vi "GVSResize Panel Child For Load.vi"(8 "spliter array":refnum<vi>[](array[refnum]), 9 "SubPanel array":refnum<vi>[](array[refnum]), 10 "DataView Array Idx":i32) -> ()   [LabVIEW 2013]
uses:
  GVSNew View Global.vi
panel:
  in  "cur_sp_hei":i32
  in  "cur_sp_wid":i32
  in  "cur_sp_ypos":i32
  in  "cur_sp_xpos":i32
  in  "sp_mUp_hei":i32
  in  "sp_mUp_wid":i32
  in  "sp_mUp_ypos":i32
  in  "sp_mUp_xpos":i32
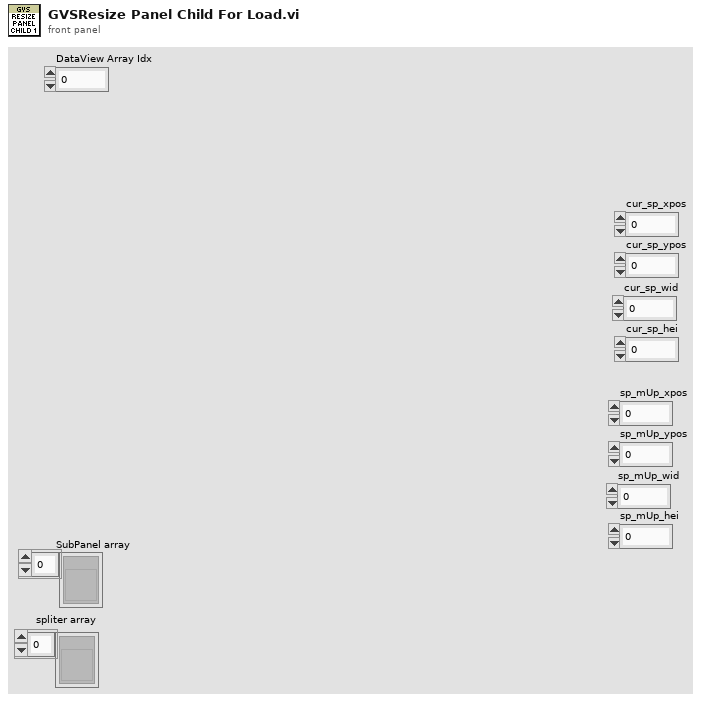
[diagram p1: front panel]
types:
  T1 = typedef "Graph Main Info Cluster.ctl" = cluster{"Selected_BarIdx":i32, "Selected_PanelIdx":i32, "Graph Main VIRef":refnum<vi>, "ToolBarClick":bool, "Spliter Ref Array":refnum<vi>[], "Panel Ref Array":refnum<vi>[], "Spliter_matrix":i32[][], "Panel_matrix":i32[][], "child_spliterIdx_matrix":i32[][], "split_pos_matrix":i32[][], "Title State":bool, "sQueueName":string, "Frame nID":i32, "Graph VIRef Array":cluster{"Graph VIRef":refnum<vi>, "Panel Idx":i32, "Frame VIRef":refnum<vi>, "Icon Ring":i32, "Graph Type":string}[], "View Type":string}
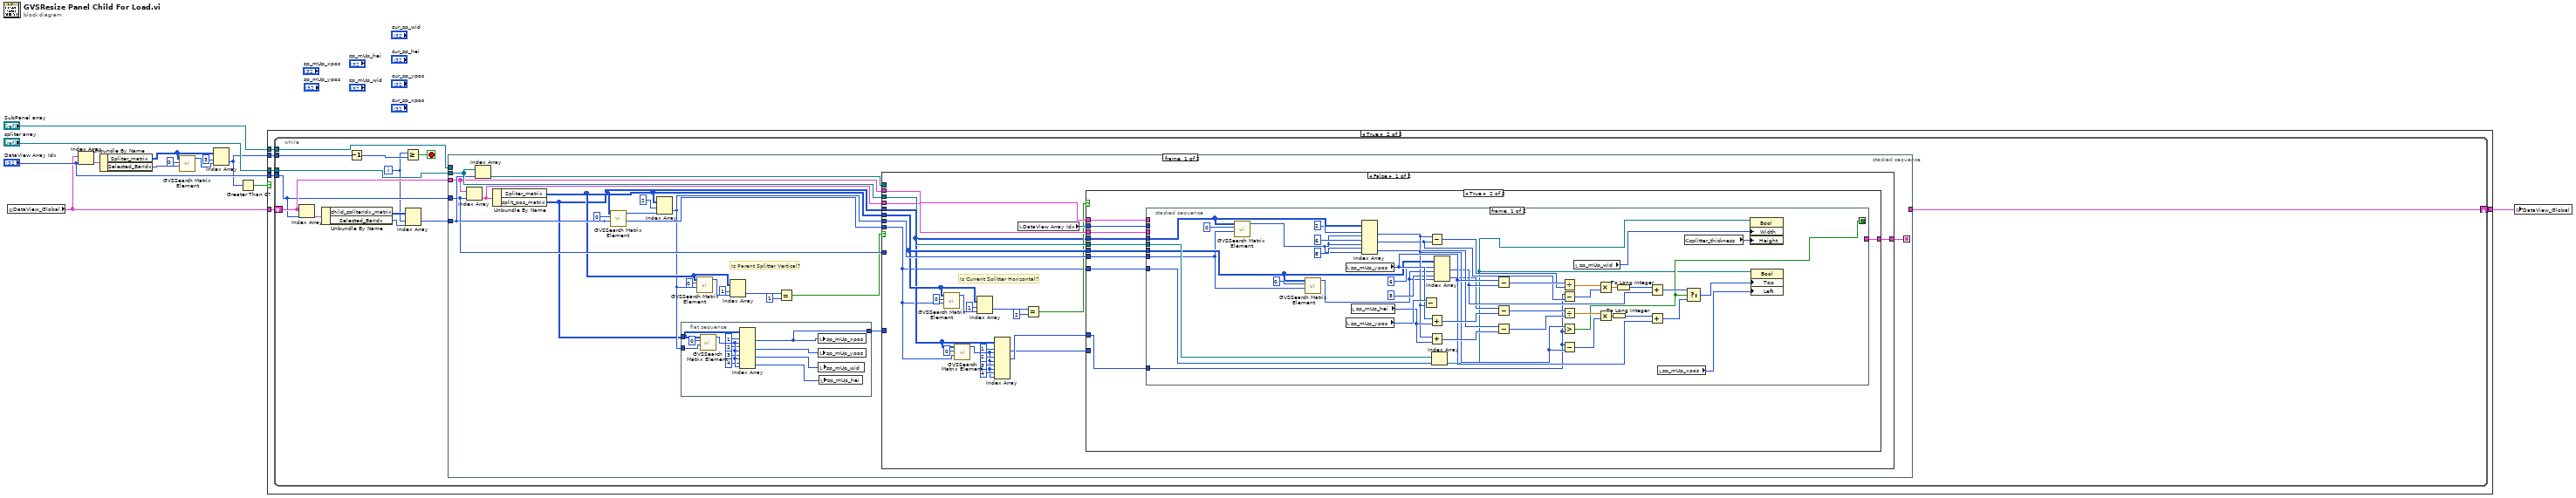
[diagram p0: block diagram]
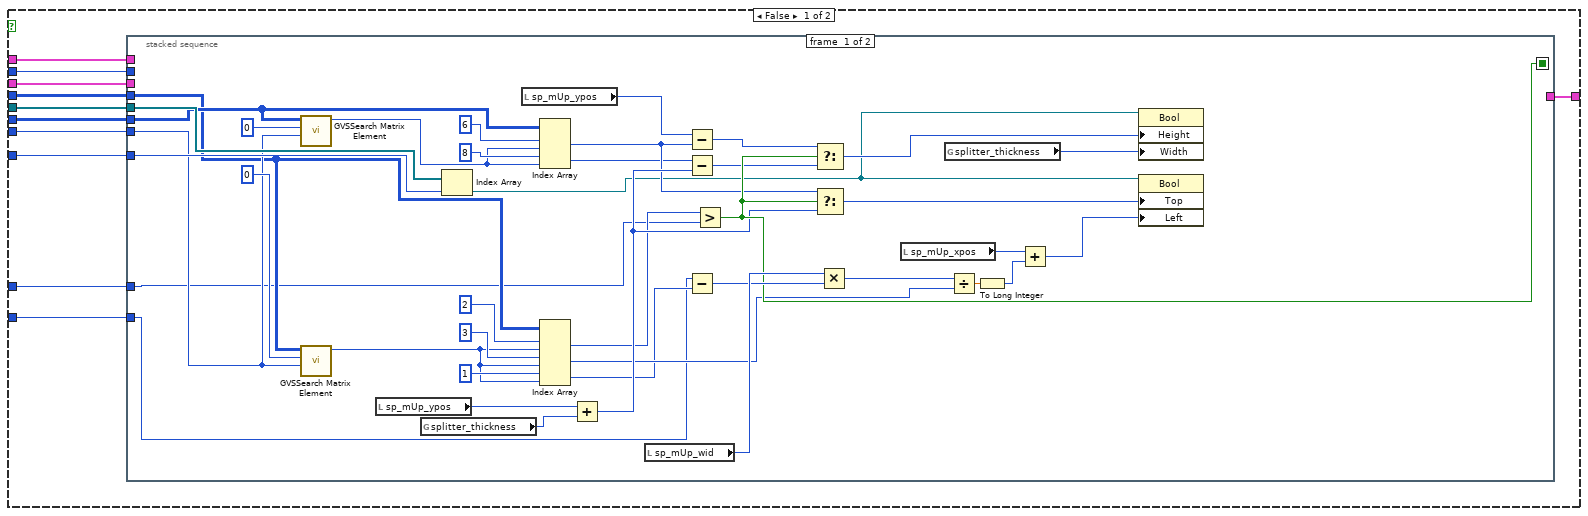
[diagram p3: hidden frame]
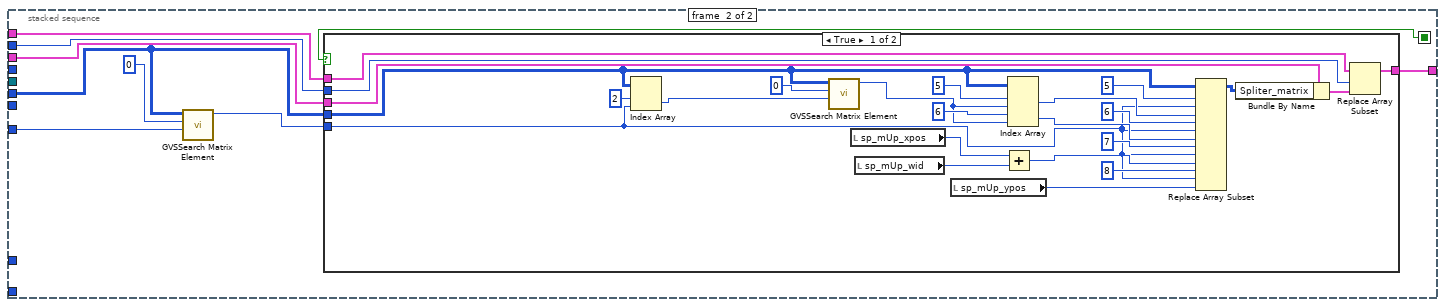
[diagram p4: hidden frame]
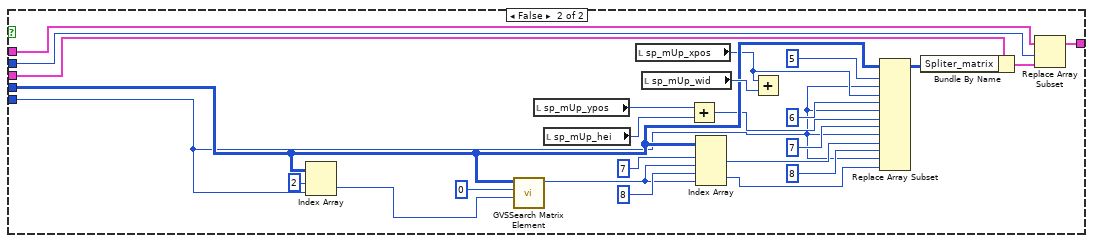
[diagram p5: hidden frame]
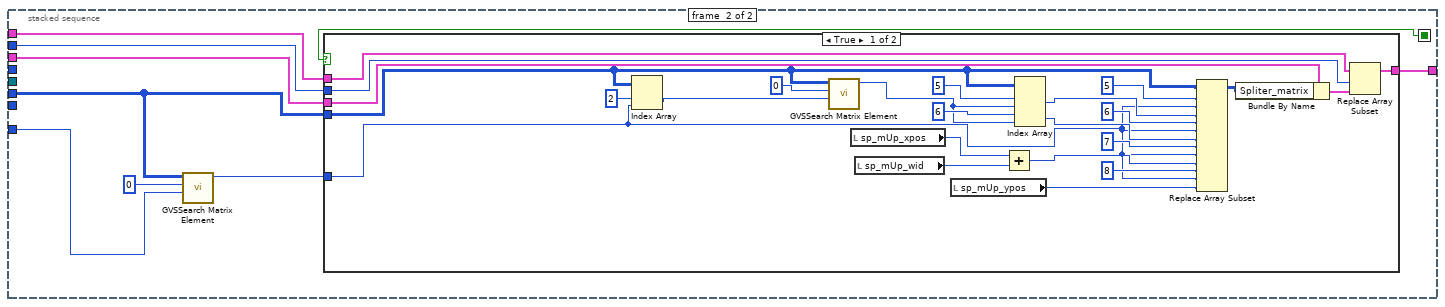
[diagram p6: hidden frame]
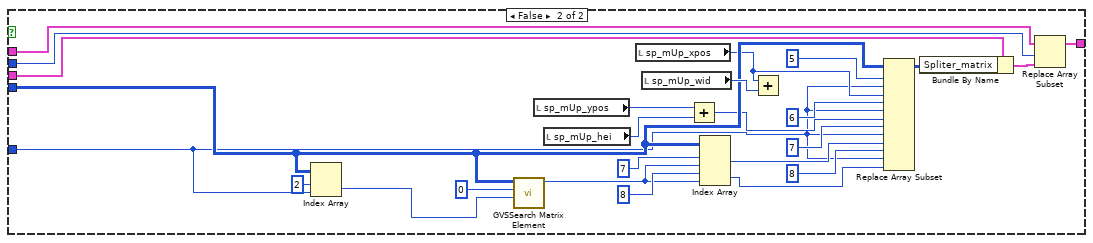
[diagram p7: hidden frame]
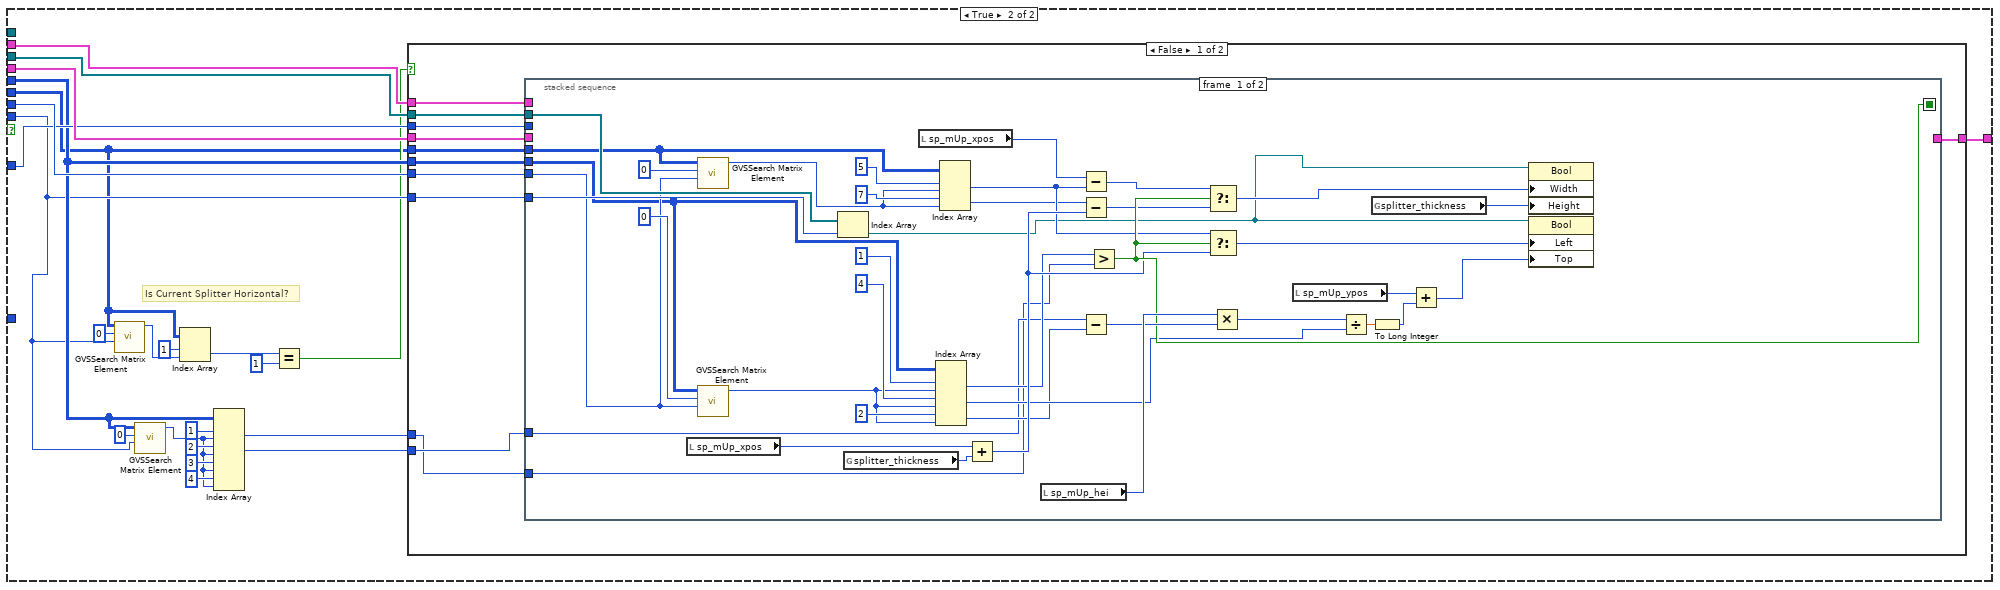
[diagram p8: hidden frame]
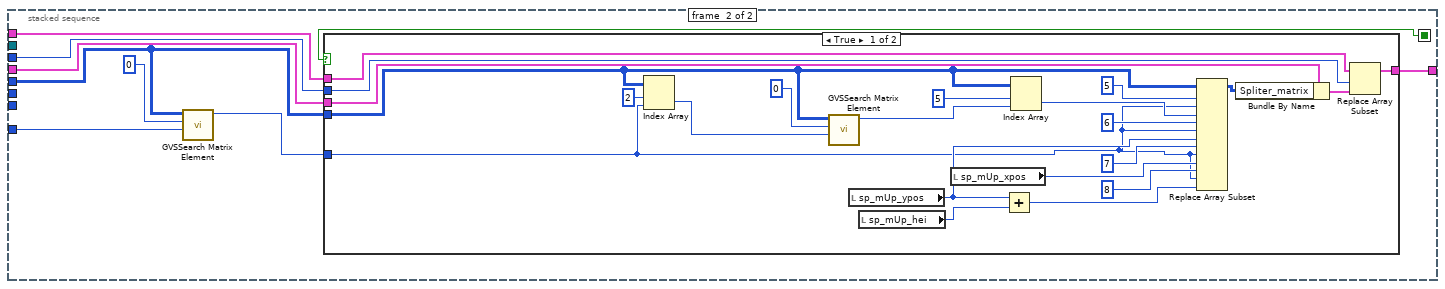
[diagram p9: hidden frame]
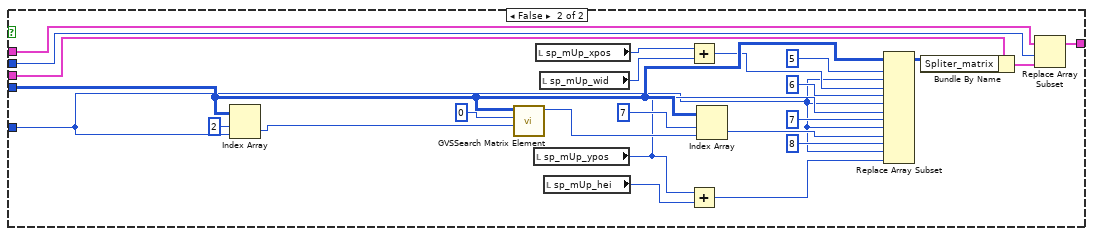
[diagram p10: hidden frame]
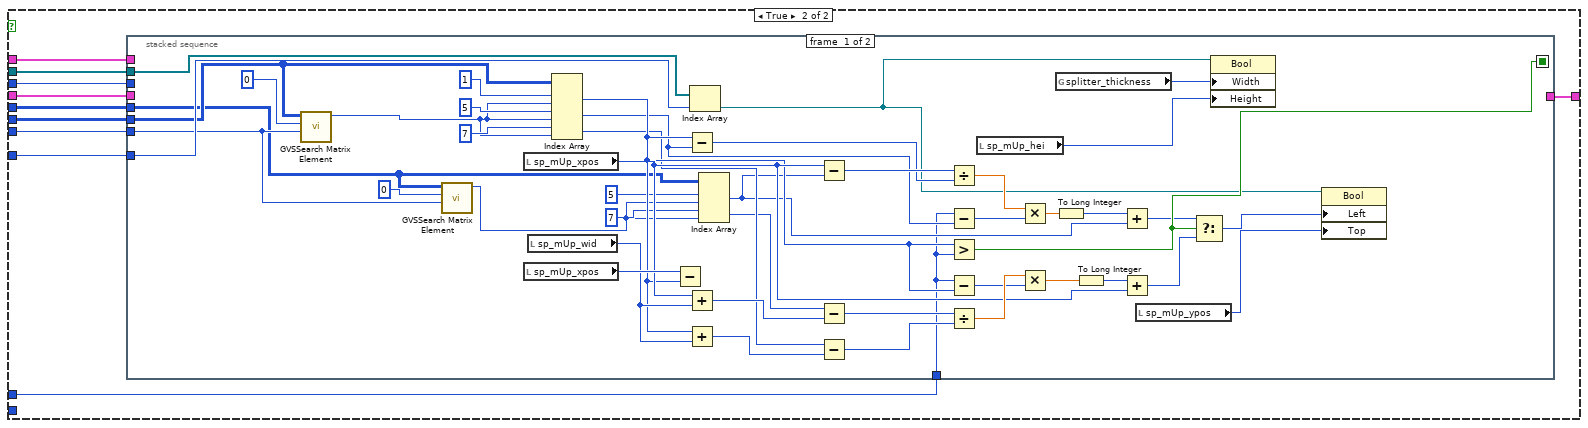
[diagram p11: hidden frame]
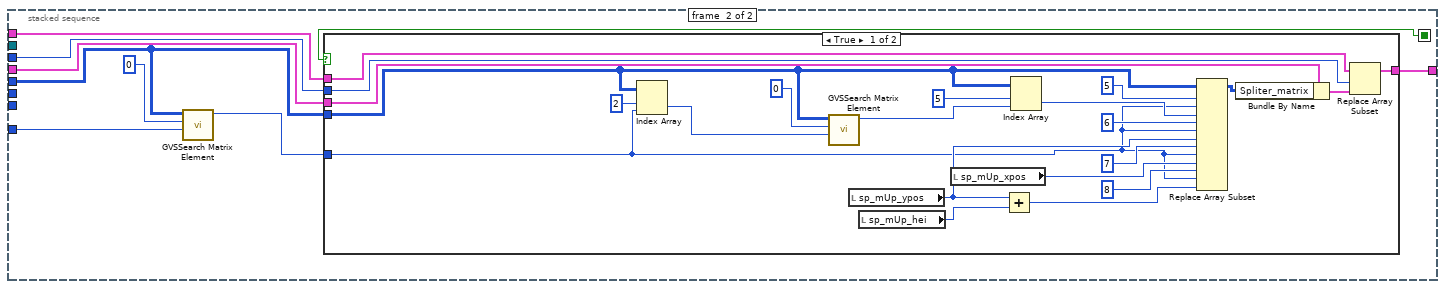
[diagram p12: hidden frame]
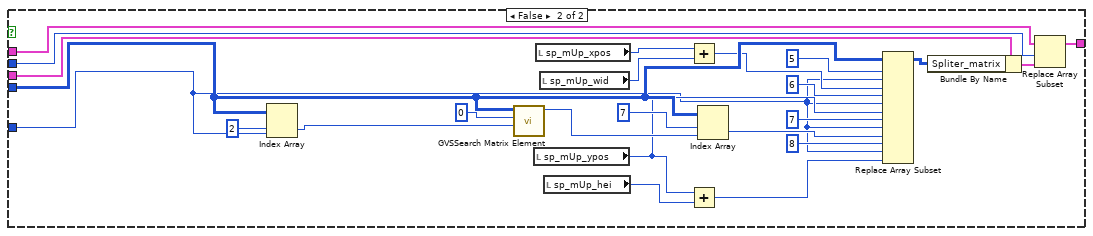
[diagram p13: hidden frame]
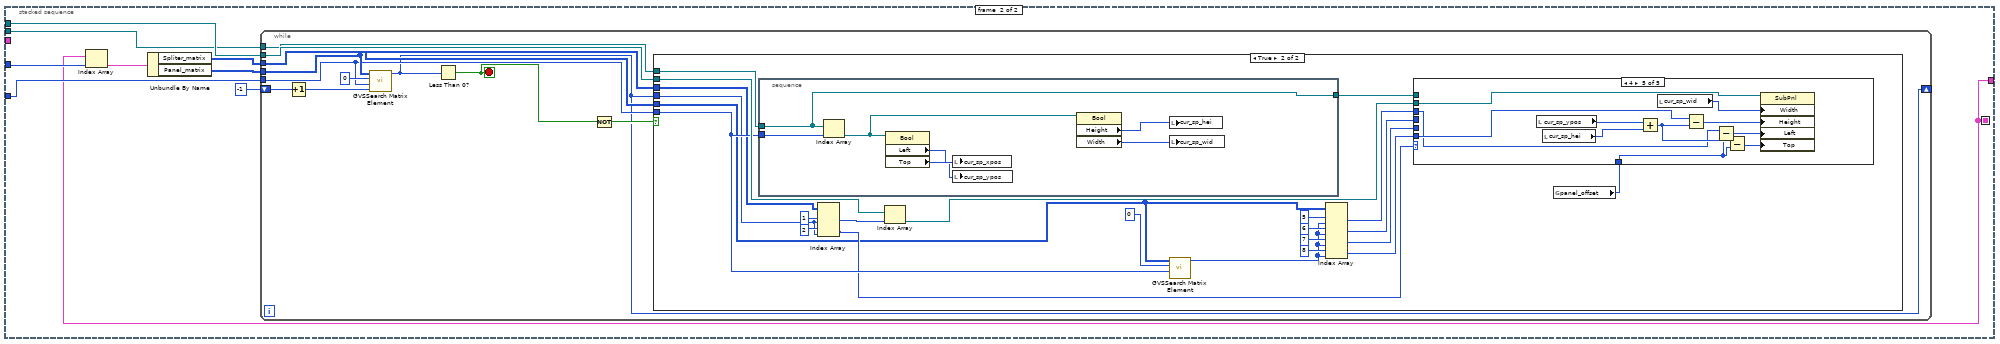
[diagram p14: hidden frame]
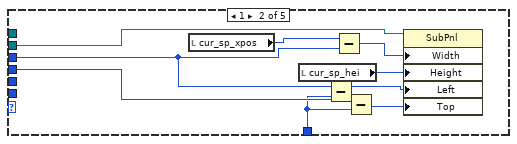
[diagram p17: hidden frame]
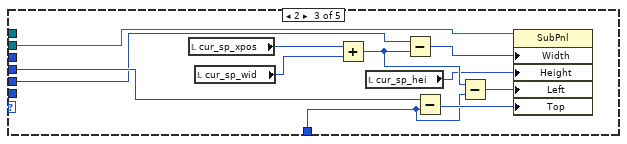
[diagram p18: hidden frame]
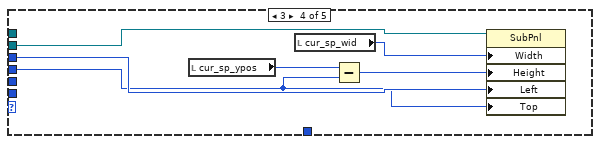
[diagram p19: hidden frame]
diagram:
  n1 = global read "GVSNew View Global.vi" "DataView_Global"() -> (w7:T1[])
  n2 = Index Array(array=w7, index="DataView Array Idx") -> (element=w10:T1)
  n3 = Unbundle By Name(w10) -> ("Spliter_matrix"=w4:i32[][], "Selected_BarIdx"=w9:i32)
  n4 = call "GVSSearch Matrix Element.vi"("element"=w9, "index (row)"=0, "matrix in"=w4) -> ("index of element"=w2:i32)  [unwired: 8 in]
  n5 = Index Array(array=w4, index (row)=3, index (col)=w2) -> (element=w1:i32)
  n6 = Greater Than 0?(x=w1) -> (x > 0?=w5:bool)
  n7 = case shown="True" w5 {
    tunnel: "spliter array" -> [_ w20]
    tunnel: "SubPanel array" -> [_ w19]
    tunnel: "DataView Array Idx" -> [_ w18]
    tunnel: w1 -> [_ w17]
    tunnel: w7 -> [w14 w16]
    tunnel: [w14 w15] -> w6
    frame False {
    }
    frame True {
      n8 = while {
        tunnel: w20 -> [w31]
        tunnel: w17 -> [w25]
        tunnel: w19 -> [w30]
        tunnel: w18 -> [w26]
        shift-right: [w27] -> w15
        shift-left: w16 -> [w28]
        i -> [w23]
        stop <- w32 stop-if-true
        n9 = Index Array(array=w28, index=w26) -> (element=w29:T1)
        n10 = Unbundle By Name(w29) -> ("child_spliterIdx_matrix"=w24:i32[][], "Selected_BarIdx"=w22:i32)
        n11 = Decrement(x=w25) -> (x-1=w33:i32)
        n12 = Greater Or Equal?(x=w23, y=w33) -> (x >= y?=w32:bool)
        n13 = Index Array(array=w24, index (row)=w23, index (col)=w22) -> (element=w21:i32)
        n14 = stacked-sequence {
          seq-local: [w47 _] -> [_ w548]
          tunnel: w31 -> [w52 w554]
          tunnel: w21 -> [w49 w556]
          tunnel: w30 -> [_ w555]
          tunnel: w26 -> [w46 w551]
          tunnel: w28 -> [w48 _]
          tunnel: [_ w548] -> w27
          frame #0 {
            # "Is Parent Splitter Vertical?"
            n15 = Index Array(array=w48, index=w46) -> (element=w51:T1)
            n16 = Index Array(array=w52, index=w49) -> (element=w53:refnum<vi>)
            n17 = Unbundle By Name(w51) -> ("Spliter_matrix"=w42:i32[][], "split_pos_matrix"=w35:i32[][])
            n18 = call "GVSSearch Matrix Element.vi"("element"=w49, "index (row)"=0, "matrix in"=w42) -> ("index of element"=w44:i32)  [unwired: 8 in]
            n19 = Index Array(array=w42, index (row)=2, index (col)=w44) -> (element=w36:i32)
            n20 = flat-sequence {
              tunnel: w36 -> [w64]
              tunnel: w35 -> [w55]
              tunnel: [w54] -> w34
              frame #0 {
                n21 = call "GVSSearch Matrix Element.vi"("element"=w64, "index (row)"=0, "matrix in"=w55) -> ("index of element"=w63:i32)  [unwired: 8 in]
                n22 = Index Array(array=w55, index (row) #1=1 ("disabled index (row)"), index (col) #1=w63, index (row) #2=2 ("disabled index (row)"), index (col) #2=w63, index (row) #3=3 ("disabled index (row)"), index (col) #3=w63, index (row) #4=4 ("disabled index (row)"), index (col) #4=w63) -> (element #1=w54:i32, element #2=w58:i32, element #3=w57:i32, element #4=w56:i32)
                n23 = local write "sp_mUp_xpos"(w54) -> ()
                n24 = local write "sp_mUp_ypos"(w58) -> ()
                n25 = local write "sp_mUp_wid"(w57) -> ()
                n26 = local write "sp_mUp_hei"(w56) -> ()
              }
            }
            n27 = call "GVSSearch Matrix Element.vi"("element"=w36, "index (row)"=0, "matrix in"=w42) -> ("index of element"=w37:i32)  [unwired: 8 in]
            n28 = Index Array(array=w42, index (row)=1 ("disabled index (row)"), index (col)=w37) -> (element=w40:i32)
            n29 = Equal?(x=w40, y=1) -> (x = y?=w38:bool)
            n30 = case shown="False" w38 {
              tunnel: w53 -> [_ _]
              tunnel: w36 -> [w88 w332]
              tunnel: w52 -> [w87 w331]
              tunnel: w49 -> [w66 w314]
              tunnel: w35 -> [w69 w315]
              tunnel: w42 -> [w77 w310]
              tunnel: w51 -> [w86 w330]
              tunnel: w48 -> [w84 w329]
              tunnel: [w83 w328] -> w47
              tunnel: w46 -> [_ w327]
              tunnel: w34 -> [_ _]
              frame False {
                # "Is Current Splitter Horizontal?"
                n31 = call "GVSSearch Matrix Element.vi"("element"=w66, "index (row)"=0, "matrix in"=w77) -> ("index of element"=w82:i32)  [unwired: 8 in]
                n32 = call "GVSSearch Matrix Element.vi"("element"=w66, "index (row)"=0, "matrix in"=w69) -> ("index of element"=w71:i32)  [unwired: 8 in]
                n33 = Index Array(array=w77, index (row)=1 ("disabled index (row)"), index (col)=w82) -> (element=w80:i32)
                n34 = Index Array(array=w69, index (row) #1=1 ("disabled index (row)"), index (col) #1=w71, index (row) #2=2 ("disabled index (row)"), index (col) #2=w71, index (row) #3=3 ("disabled index (row)"), index (col) #3=w71, index (row) #4=4 ("disabled index (row)"), index (col) #4=w71) -> (element #1=w67:i32, element #2=w68:i32)  [unwired: 2 out]
                n35 = local read "DataView Array Idx"() -> (w85:i32)
                n36 = Equal?(x=w80, y=2) -> (x = y?=w76:bool)
                n37 = case shown="True" w76 {
                  tunnel: w88 -> [w97 w204]
                  tunnel: w87 -> [w99 w205]
                  tunnel: w66 -> [w98 w206]
                  tunnel: w69 -> [w96 w203]
                  tunnel: w77 -> [w95 w202]
                  tunnel: w86 -> [w94 w201]
                  tunnel: w85 -> [w93 w200]
                  tunnel: w84 -> [w92 w199]
                  tunnel: [w91 w198] -> w83
                  tunnel: w68 -> [w90 w197]
                  tunnel: w67 -> [w89 _]
                  frame False {
                    n38 = stacked-sequence {
                      seq-local: [w127 _] -> [_ w147]
                      tunnel: w99 -> [w138 _]
                      tunnel: w98 -> [w137 w142]
                      tunnel: w97 -> [w120 _]
                      tunnel: w96 -> [w113 _]
                      tunnel: w95 -> [w119 w144]
                      tunnel: w94 -> [_ w146]
                      tunnel: w93 -> [_ w145]
                      tunnel: w92 -> [_ w140]
                      tunnel: [_ w139] -> w91
                      tunnel: w90 -> [w105 _]
                      tunnel: w89 -> [w104 _]
                      frame #0 {
                        n39 = call "GVSSearch Matrix Element.vi"("element"=w120, "index (row)"=0, "matrix in"=w119) -> ("index of element"=w116:i32)  [unwired: 8 in]
                        n40 = call "GVSSearch Matrix Element.vi"("element"=w120, "index (row)"=0, "matrix in"=w113) -> ("index of element"=w109:i32)  [unwired: 8 in]
                        n41 = local read "sp_mUp_ypos"() -> (w136:i32)
                        n42 = global read "GVSNew View Global.vi" "splitter_thickness"() -> (w100:u32)
                        n43 = Index Array(array=w138, index=w137) -> (element=w103:refnum<vi>)
                        n44 = local read "sp_mUp_ypos"() -> (w126:i32)
                        n45 = Index Array(array=w119, index (row) #1=6 ("index (row)"), index (col) #1=w116, index (row) #2=8 ("index (row)"), index (col) #2=w116) -> (element #1=w115:i32, element #2=w114:i32)
                        n46 = Index Array(array=w113, index (row) #1=2 ("index (row)"), index (col) #1=w109, index (row) #2=3 ("index (row)"), index (col) #2=w109, index (row) #3=1 ("index (row)"), index (col) #3=w109) -> (element #1=w108:i32, element #2=w107:i32, element #3=w106:i32)
                        n47 = Add(x=w136, y=w100) -> (x+y=w124:u32)
                        n48 = local read "sp_mUp_wid"() -> (w133:i32)
                        n49 = Subtract(x=w126, y=w115) -> (x-y=w125:i32)
                        n50 = Subtract(x=w114, y=w124) -> (x-y=w123:u32)
                        n51 = Subtract(x=w104, y=w106) -> (x-y=w128:i32)
                        n52 = Greater?(x=w108, y=w105) -> (0:w127:bool)
                        n53 = Select(t=w125, s=w127, f=w123) -> (s? t:f=w134:u32)
                        n54 = Select(t=w115, s=w127, f=w124) -> (s? t:f=w135:u32)
                        n55 = Multiply(x=w133, y=w128) -> (x*y=w132:i32)
                        n56 = local read "sp_mUp_xpos"() -> (w131:i32)
                        n57 = global read "GVSNew View Global.vi" "splitter_thickness"() -> (w102:u32)
                        n58 = Divide(x=w132, y=w107) -> (x/y=w130:dbl)
                        n59 = To Long Integer(number=w130) -> (32bit integer=w101:i32)
                        n60 = Add(x=w131, y=w101) -> (x+y=w129:i32)
                        n61 = property class="Bool"(reference=w103, "Height"=w134, "Width"=w102) -> ()  [unwired: 1 in, 2 out]
                        n62 = property class="Bool"(reference=w103, "Top"=w135, "Left"=w129) -> ()  [unwired: 1 in, 2 out]
                      }
                      frame #1 {
                        n63 = call "GVSSearch Matrix Element.vi"("element"=w142, "index (row)"=0, "matrix in"=w144) -> ("index of element"=w141:i32)  [unwired: 8 in]
                        n64 = case shown="True" w147 {
                          tunnel: w141 -> [w150 w174]
                          tunnel: w144 -> [w158 w182]
                          tunnel: w146 -> [w168 w192]
                          tunnel: w145 -> [w167 w191]
                          tunnel: w140 -> [w165 w189]
                          tunnel: [w164 w188] -> w139
                          frame True {
                            n65 = Index Array(array=w158, index (row)=2, index (col)=w150) -> (element=w162:i32)
                            n66 = call "GVSSearch Matrix Element.vi"("element"=w162, "index (row)"=0, "matrix in"=w158) -> ("index of element"=w159:i32)  [unwired: 8 in]
                            n67 = local read "sp_mUp_xpos"() -> (w170:i32)
                            n68 = local read "sp_mUp_wid"() -> (w171:i32)
                            n69 = local read "sp_mUp_ypos"() -> (w149:i32)
                            n70 = Add(x=w170, y=w171) -> (x+y=w152:i32)
                            n71 = Index Array(array=w158, index (row) #1=5 ("index (row)"), index (col) #1=w159, index (row) #2=6 ("index (row)"), index (col) #2=w159) -> (element #1=w156:i32, element #2=w154:i32)
                            n72 = Replace Array Subset(array=w158, new element #1=w156, index (row) #1=5 ("disabled index (row)"), index (col) #1=w150, new element #2=w154, index (row) #2=6 ("disabled index (row)"), index (col) #2=w150, new element #3=w152, index (row) #3=7 ("disabled index (row)"), index (col) #3=w150, new element #4=w149, index (row) #4=8 ("disabled index (row)"), index (col) #4=w150) -> (w148:i32[][])
                            n73 = Bundle By Name(cluster=w168, "Spliter_matrix"=w148) -> (w169:T1)
                            n74 = Replace Array Subset(array=w165, new element=w169, index=w167) -> (w164:T1[])
                          }
                          frame False {
                            n75 = Index Array(array=w182, index (row)=2, index (col)=w174) -> (element=w186:i32)
                            n76 = call "GVSSearch Matrix Element.vi"("element"=w186, "index (row)"=0, "matrix in"=w182) -> ("index of element"=w183:i32)  [unwired: 8 in]
                            n77 = local read "sp_mUp_ypos"() -> (w195:i32)
                            n78 = local read "sp_mUp_hei"() -> (w196:i32)
                            n79 = local read "sp_mUp_xpos"() -> (w180:i32)
                            n80 = local read "sp_mUp_wid"() -> (w194:i32)
                            n81 = Add(x=w195, y=w196) -> (x+y=w178:i32)
                            n82 = Index Array(array=w182, index (row) #1=7 ("index (row)"), index (col) #1=w183, index (row) #2=8 ("index (row)"), index (col) #2=w183) -> (element #1=w176:i32, element #2=w173:i32)
                            n83 = Add(x=w180, y=w194) -> ()  [unwired: 1 out]
                            n84 = Replace Array Subset(array=w182, new element #1=w180, index (row) #1=5 ("disabled index (row)"), index (col) #1=w174, new element #2=w178, index (row) #2=6 ("disabled index (row)"), index (col) #2=w174, new element #3=w176, index (row) #3=7 ("disabled index (row)"), index (col) #3=w174, new element #4=w173, index (row) #4=8 ("disabled index (row)"), index (col) #4=w174) -> (w172:i32[][])
                            n85 = Bundle By Name(cluster=w192, "Spliter_matrix"=w172) -> (w193:T1)
                            n86 = Replace Array Subset(array=w189, new element=w193, index=w191) -> (w188:T1[])
                          }
                        }
                      }
                    }
                  }
                  frame True {
                    n87 = stacked-sequence {
                      seq-local: [w230 _] -> [_ w260]
                      tunnel: w206 -> [w213 w256]
                      tunnel: w205 -> [w250 _]
                      tunnel: w204 -> [w211 _]
                      tunnel: w203 -> [w227 _]
                      tunnel: w202 -> [w219 w255]
                      tunnel: w201 -> [_ w259]
                      tunnel: w200 -> [_ w258]
                      tunnel: w199 -> [_ w253]
                      tunnel: [_ w252] -> w198
                      tunnel: w197 -> [w212 _]
                      frame #0 {
                        n88 = call "GVSSearch Matrix Element.vi"("element"=w211, "index (row)"=0, "matrix in"=w227) -> ("index of element"=w223:i32)  [unwired: 8 in]
                        n89 = call "GVSSearch Matrix Element.vi"("element"=w211, "index (row)"=0, "matrix in"=w219) -> ("index of element"=w216:i32)  [unwired: 8 in]
                        n90 = local read "sp_mUp_ypos"() -> (w234:i32)
                        n91 = local read "sp_mUp_ypos"() -> (w251:i32)
                        n92 = local read "sp_mUp_hei"() -> (w247:i32)
                        n93 = Index Array(array=w227, index (row) #1=2 ("index (row)"), index (col) #1=w223, index (row) #2=6 ("index (row)"), index (col) #2=w223, index (row) #3=8 ("index (row)"), index (col) #3=w223) -> (element #1=w222:i32, element #2=w221:i32, element #3=w220:i32)
                        n94 = Subtract(x=w251, y=w222) -> ()  [unwired: 1 out]
                        n95 = Subtract(x=w222, y=w221) -> (x-y=w241:i32)
                        n96 = Add(x=w234, y=w247) -> (x+y=w235:i32)
                        n97 = Add(x=w222, y=w247) -> (x+y=w236:i32)
                        n98 = Index Array(array=w250, index=w213) -> (element=w210:refnum<vi>)
                        n99 = Index Array(array=w219, index (row) #1=6 ("index (row)"), index (col) #1=w216, index (row) #2=8 ("index (row)"), index (col) #2=w216) -> (element #1=w215:i32, element #2=w214:i32)
                        n100 = Subtract(x=w234, y=w215) -> (x-y=w242:i32)
                        n101 = Subtract(x=w214, y=w235) -> (x-y=w246:i32)
                        n102 = Subtract(x=w220, y=w236) -> (x-y=w245:i32)
                        n103 = Divide(x=w242, y=w241) -> (x/y=w240:dbl)
                        n104 = Subtract(x=w212, y=w221) -> (x-y=w239:i32)
                        n105 = Divide(x=w246, y=w245) -> (x/y=w244:dbl)
                        n106 = Greater?(x=w222, y=w212) -> (0:w230:bool)
                        n107 = Subtract(x=w212, y=w222) -> (x-y=w237:i32)
                        n108 = local read "sp_mUp_wid"() -> (w249:i32)
                        n109 = Multiply(x=w240, y=w239) -> (x*y=w238:dbl)
                        n110 = Multiply(x=w244, y=w237) -> (x*y=w243:dbl)
                        n111 = To Long Integer(number=w243) -> (32bit integer=w208:i32)
                        n112 = To Long Integer(number=w238) -> (32bit integer=w209:i32)
                        n113 = Add(x=w209, y=w215) -> (x+y=w233:i32)
                        n114 = Add(x=w208, y=w234) -> (x+y=w232:i32)
                        n115 = local read "sp_mUp_xpos"() -> (w248:i32)
                        n116 = global read "GVSNew View Global.vi" "splitter_thickness"() -> (w207:u32)
                        n117 = Select(t=w233, s=w230, f=w232) -> (s? t:f=w231:i32)
                        n118 = property class="Bool"(reference=w210, "Width"=w249, "Height"=w207) -> ()  [unwired: 1 in, 2 out]
                        n119 = property class="Bool"(reference=w210, "Top"=w231, "Left"=w248) -> ()  [unwired: 1 in, 2 out]
                      }
                      frame #1 {
                        n120 = call "GVSSearch Matrix Element.vi"("element"=w256, "index (row)"=0, "matrix in"=w255) -> ("index of element"=w254:i32)  [unwired: 8 in]
                        n121 = case shown="True" w260 {
                          tunnel: w254 -> [w262 w286]
                          tunnel: w255 -> [w271 w295]
                          tunnel: w259 -> [w281 w305]
                          tunnel: w258 -> [w280 w304]
                          tunnel: w253 -> [w278 w302]
                          tunnel: [w277 w301] -> w252
                          frame True {
                            n122 = Index Array(array=w271, index (row)=2, index (col)=w262) -> (element=w276:i32)
                            n123 = call "GVSSearch Matrix Element.vi"("element"=w276, "index (row)"=0, "matrix in"=w271) -> ("index of element"=w272:i32)  [unwired: 8 in]
                            n124 = local read "sp_mUp_xpos"() -> (w283:i32)
                            n125 = local read "sp_mUp_wid"() -> (w284:i32)
                            n126 = local read "sp_mUp_ypos"() -> (w261:i32)
                            n127 = Add(x=w283, y=w284) -> (x+y=w264:i32)
                            n128 = Index Array(array=w271, index (row) #1=5 ("index (row)"), index (col) #1=w272, index (row) #2=6 ("index (row)"), index (col) #2=w272) -> (element #1=w268:i32, element #2=w266:i32)
                            n129 = Replace Array Subset(array=w271, new element #1=w268, index (row) #1=5 ("disabled index (row)"), index (col) #1=w262, new element #2=w266, index (row) #2=6 ("disabled index (row)"), index (col) #2=w262, new element #3=w264, index (row) #3=7 ("disabled index (row)"), index (col) #3=w262, new element #4=w261, index (row) #4=8 ("disabled index (row)"), index (col) #4=w262) -> (w270:i32[][])
                            n130 = Bundle By Name(cluster=w281, "Spliter_matrix"=w270) -> (w282:T1)
                            n131 = Replace Array Subset(array=w278, new element=w282, index=w280) -> (w277:T1[])
                          }
                          frame False {
                            n132 = Index Array(array=w295, index (row)=2, index (col)=w286) -> (element=w299:i32)
                            n133 = call "GVSSearch Matrix Element.vi"("element"=w299, "index (row)"=0, "matrix in"=w295) -> ("index of element"=w296:i32)  [unwired: 8 in]
                            n134 = local read "sp_mUp_ypos"() -> (w308:i32)
                            n135 = local read "sp_mUp_hei"() -> (w309:i32)
                            n136 = local read "sp_mUp_xpos"() -> (w292:i32)
                            n137 = local read "sp_mUp_wid"() -> (w307:i32)
                            n138 = Add(x=w308, y=w309) -> (x+y=w290:i32)
                            n139 = Index Array(array=w295, index (row) #1=7 ("index (row)"), index (col) #1=w296, index (row) #2=8 ("index (row)"), index (col) #2=w296) -> (element #1=w288:i32, element #2=w285:i32)
                            n140 = Add(x=w292, y=w307) -> ()  [unwired: 1 out]
                            n141 = Replace Array Subset(array=w295, new element #1=w292, index (row) #1=5 ("disabled index (row)"), index (col) #1=w286, new element #2=w290, index (row) #2=6 ("disabled index (row)"), index (col) #2=w286, new element #3=w288, index (row) #3=7 ("disabled index (row)"), index (col) #3=w286, new element #4=w285, index (row) #4=8 ("disabled index (row)"), index (col) #4=w286) -> (w294:i32[][])
                            n142 = Bundle By Name(cluster=w305, "Spliter_matrix"=w294) -> (w306:T1)
                            n143 = Replace Array Subset(array=w302, new element=w306, index=w304) -> (w301:T1[])
                          }
                        }
                      }
                    }
                  }
                }
              }
              frame True {
                # "Is Current Splitter Horizontal?"
                n144 = call "GVSSearch Matrix Element.vi"("element"=w314, "index (row)"=0, "matrix in"=w310) -> ("index of element"=w326:i32)  [unwired: 8 in]
                n145 = call "GVSSearch Matrix Element.vi"("element"=w314, "index (row)"=0, "matrix in"=w315) -> ("index of element"=w317:i32)  [unwired: 8 in]
                n146 = Index Array(array=w310, index (row)=1 ("disabled index (row)"), index (col)=w326) -> (element=w324:i32)
                n147 = Index Array(array=w315, index (row) #1=1 ("disabled index (row)"), index (col) #1=w317, index (row) #2=2 ("disabled index (row)"), index (col) #2=w317, index (row) #3=3 ("disabled index (row)"), index (col) #3=w317, index (row) #4=4 ("disabled index (row)"), index (col) #4=w317) -> (element #1=w312:i32, element #2=w311:i32)  [unwired: 2 out]
                n148 = Equal?(x=w324, y=1) -> (x = y?=w313:bool)
                n149 = case shown="False" w313 {
                  tunnel: w332 -> [w342 w447]
                  tunnel: w331 -> [w343 w446]
                  tunnel: w314 -> [w341 w445]
                  tunnel: w315 -> [w340 w444]
                  tunnel: w310 -> [w339 w443]
                  tunnel: w330 -> [w338 w442]
                  tunnel: w327 -> [w337 w441]
                  tunnel: w329 -> [w336 w440]
                  tunnel: [w335 w439] -> w328
                  tunnel: w312 -> [w333 w438]
                  tunnel: w311 -> [w334 _]
                  frame False {
                    n150 = stacked-sequence {
                      seq-local: [w371 _] -> [_ w391]
                      tunnel: w343 -> [w382 _]
                      tunnel: w342 -> [w364 _]
                      tunnel: w341 -> [w381 w386]
                      tunnel: w340 -> [w363 _]
                      tunnel: w339 -> [w355 w388]
                      tunnel: w338 -> [_ w390]
                      tunnel: w337 -> [_ w389]
                      tunnel: w336 -> [_ w384]
                      tunnel: [_ w383] -> w335
                      tunnel: w334 -> [w349 _]
                      tunnel: w333 -> [w348 _]
                      frame #0 {
                        n151 = local read "sp_mUp_xpos"() -> (w380:i32)
                        n152 = call "GVSSearch Matrix Element.vi"("element"=w364, "index (row)"=0, "matrix in"=w355) -> ("index of element"=w352:i32)  [unwired: 8 in]
                        n153 = call "GVSSearch Matrix Element.vi"("element"=w364, "index (row)"=0, "matrix in"=w363) -> ("index of element"=w359:i32)  [unwired: 8 in]
                        n154 = Index Array(array=w382, index=w381) -> (element=w347:refnum<vi>)
                        n155 = global read "GVSNew View Global.vi" "splitter_thickness"() -> (w344:u32)
                        n156 = local read "sp_mUp_xpos"() -> (w370:i32)
                        n157 = Index Array(array=w363, index (row) #1=1 ("index (row)"), index (col) #1=w359, index (row) #2=4 ("index (row)"), index (col) #2=w359, index (row) #3=2 ("index (row)"), index (col) #3=w359) -> (element #1=w358:i32, element #2=w357:i32, element #3=w356:i32)
                        n158 = Index Array(array=w355, index (row) #1=5 ("index (row)"), index (col) #1=w352, index (row) #2=7 ("index (row)"), index (col) #2=w352) -> (element #1=w351:i32, element #2=w350:i32)
                        n159 = Add(x=w380, y=w344) -> (x+y=w368:u32)
                        n160 = local read "sp_mUp_hei"() -> (w378:i32)
                        n161 = Subtract(x=w370, y=w351) -> (x-y=w369:i32)
                        n162 = Subtract(x=w350, y=w368) -> (x-y=w367:u32)
                        n163 = Subtract(x=w349, y=w356) -> (x-y=w377:i32)
                        n164 = Greater?(x=w358, y=w348) -> (0:w371:bool)
                        n165 = Select(t=w369, s=w371, f=w367) -> (s? t:f=w372:u32)
                        n166 = Select(t=w351, s=w371, f=w368) -> (s? t:f=w379:u32)
                        n167 = Multiply(x=w378, y=w377) -> (x*y=w376:i32)
                        n168 = local read "sp_mUp_ypos"() -> (w375:i32)
                        n169 = Divide(x=w376, y=w357) -> (x/y=w374:dbl)
                        n170 = global read "GVSNew View Global.vi" "splitter_thickness"() -> (w346:u32)
                        n171 = To Long Integer(number=w374) -> (32bit integer=w345:i32)
                        n172 = Add(x=w375, y=w345) -> (x+y=w373:i32)
                        n173 = property class="Bool"(reference=w347, "Width"=w372, "Height"=w346) -> ()  [unwired: 1 in, 2 out]
                        n174 = property class="Bool"(reference=w347, "Left"=w379, "Top"=w373) -> ()  [unwired: 1 in, 2 out]
                      }
                      frame #1 {
                        n175 = call "GVSSearch Matrix Element.vi"("element"=w386, "index (row)"=0, "matrix in"=w388) -> ("index of element"=w385:i32)  [unwired: 8 in]
                        n176 = case shown="True" w391 {
                          tunnel: w385 -> [w393 w416]
                          tunnel: w388 -> [w402 w424]
                          tunnel: w390 -> [w411 w433]
                          tunnel: w389 -> [w410 w432]
                          tunnel: w384 -> [w408 w430]
                          tunnel: [w407 w429] -> w383
                          frame True {
                            n177 = Index Array(array=w402, index (row)=2, index (col)=w393) -> (element=w405:i32)
                            n178 = call "GVSSearch Matrix Element.vi"("element"=w405, "index (row)"=0, "matrix in"=w402) -> ("index of element"=w403:i32)  [unwired: 8 in]
                            n179 = local read "sp_mUp_ypos"() -> (w398:i32)
                            n180 = local read "sp_mUp_hei"() -> (w413:i32)
                            n181 = local read "sp_mUp_xpos"() -> (w396:i32)
                            n182 = Add(x=w398, y=w413) -> (x+y=w394:i32)
                            n183 = Index Array(array=w402, index (row)=5, index (col)=w403) -> (element=w400:i32)
                            n184 = Replace Array Subset(array=w402, new element #1=w400, index (row) #1=5 ("disabled index (row)"), index (col) #1=w393, new element #2=w398, index (row) #2=6 ("disabled index (row)"), index (col) #2=w393, new element #3=w396, index (row) #3=7 ("disabled index (row)"), index (col) #3=w393, new element #4=w394, index (row) #4=8 ("disabled index (row)"), index (col) #4=w393) -> (w392:i32[][])
                            n185 = Bundle By Name(cluster=w411, "Spliter_matrix"=w392) -> (w412:T1)
                            n186 = Replace Array Subset(array=w408, new element=w412, index=w410) -> (w407:T1[])
                          }
                          frame False {
                            n187 = Index Array(array=w424, index (row)=2, index (col)=w416) -> (element=w427:i32)
                            n188 = call "GVSSearch Matrix Element.vi"("element"=w427, "index (row)"=0, "matrix in"=w424) -> ("index of element"=w425:i32)  [unwired: 8 in]
                            n189 = local read "sp_mUp_ypos"() -> (w420:i32)
                            n190 = local read "sp_mUp_xpos"() -> (w436:i32)
                            n191 = local read "sp_mUp_wid"() -> (w435:i32)
                            n192 = local read "sp_mUp_hei"() -> (w437:i32)
                            n193 = Add(x=w436, y=w435) -> (x+y=w422:i32)
                            n194 = Add(x=w420, y=w437) -> (x+y=w415:i32)
                            n195 = Index Array(array=w424, index (row)=7, index (col)=w425) -> (element=w418:i32)
                            n196 = Replace Array Subset(array=w424, new element #1=w422, index (row) #1=5 ("disabled index (row)"), index (col) #1=w416, new element #2=w420, index (row) #2=6 ("disabled index (row)"), index (col) #2=w416, new element #3=w418, index (row) #3=7 ("disabled index (row)"), index (col) #3=w416, new element #4=w415, index (row) #4=8 ("disabled index (row)"), index (col) #4=w416) -> (w414:i32[][])
                            n197 = Bundle By Name(cluster=w433, "Spliter_matrix"=w414) -> (w434:T1)
                            n198 = Replace Array Subset(array=w430, new element=w434, index=w432) -> (w429:T1[])
                          }
                        }
                      }
                    }
                  }
                  frame True {
                    n199 = stacked-sequence {
                      seq-local: [w487 _] -> [_ w501]
                      tunnel: w447 -> [w467 _]
                      tunnel: w446 -> [w492 _]
                      tunnel: w445 -> [w474 w496]
                      tunnel: w444 -> [w466 _]
                      tunnel: w443 -> [w458 w497]
                      tunnel: w442 -> [_ w500]
                      tunnel: w441 -> [_ w499]
                      tunnel: w440 -> [_ w494]
                      tunnel: [_ w493] -> w439
                      tunnel: w438 -> [w452 _]
                      frame #0 {
                        n200 = call "GVSSearch Matrix Element.vi"("element"=w467, "index (row)"=0, "matrix in"=w466) -> ("index of element"=w462:i32)  [unwired: 8 in]
                        n201 = call "GVSSearch Matrix Element.vi"("element"=w467, "index (row)"=0, "matrix in"=w458) -> ("index of element"=w455:i32)  [unwired: 8 in]
                        n202 = local read "sp_mUp_xpos"() -> (w470:i32)
                        n203 = local read "sp_mUp_xpos"() -> (w490:i32)
                        n204 = local read "sp_mUp_wid"() -> (w486:i32)
                        n205 = Index Array(array=w466, index (row) #1=1 ("index (row)"), index (col) #1=w462, index (row) #2=5 ("index (row)"), index (col) #2=w462, index (row) #3=7 ("index (row)"), index (col) #3=w462) -> (element #1=w461:i32, element #2=w460:i32, element #3=w459:i32)
                        n206 = Subtract(x=w490, y=w461) -> ()  [unwired: 1 out]
                        n207 = Subtract(x=w461, y=w460) -> (x-y=w479:i32)
                        n208 = Add(x=w470, y=w486) -> (x+y=w471:i32)
                        n209 = Add(x=w461, y=w486) -> (x+y=w472:i32)
                        n210 = Index Array(array=w492, index=w474) -> (element=w451:refnum<vi>)
                        n211 = Index Array(array=w458, index (row) #1=5 ("index (row)"), index (col) #1=w455, index (row) #2=7 ("index (row)"), index (col) #2=w455) -> (element #1=w453:i32, element #2=w454:i32)
                        n212 = Subtract(x=w470, y=w453) -> (x-y=w480:i32)
                        n213 = Subtract(x=w454, y=w471) -> (x-y=w485:i32)
                        n214 = Subtract(x=w459, y=w472) -> (x-y=w484:i32)
                        n215 = Divide(x=w480, y=w479) -> (x/y=w478:dbl)
                        n216 = Subtract(x=w452, y=w460) -> (x-y=w477:i32)
                        n217 = Greater?(x=w461, y=w452) -> (0:w487:bool)
                        n218 = Subtract(x=w452, y=w461) -> (x-y=w473:i32)
                        n219 = Divide(x=w485, y=w484) -> (x/y=w483:dbl)
                        n220 = local read "sp_mUp_hei"() -> (w491:i32)
                        n221 = Multiply(x=w478, y=w477) -> (x*y=w476:dbl)
                        n222 = Multiply(x=w483, y=w473) -> (x*y=w482:dbl)
                        n223 = global read "GVSNew View Global.vi" "splitter_thickness"() -> (w448:u32)
                        n224 = To Long Integer(number=w476) -> (32bit integer=w450:i32)
                        n225 = To Long Integer(number=w482) -> (32bit integer=w449:i32)
                        n226 = Add(x=w450, y=w453) -> (x+y=w475:i32)
                        n227 = Add(x=w449, y=w470) -> (x+y=w481:i32)
                        n228 = local read "sp_mUp_ypos"() -> (w489:i32)
                        n229 = Select(t=w475, s=w487, f=w481) -> (s? t:f=w488:i32)
                        n230 = property class="Bool"(reference=w451, "Width"=w448, "Height"=w491) -> ()  [unwired: 1 in, 2 out]
                        n231 = property class="Bool"(reference=w451, "Left"=w488, "Top"=w489) -> ()  [unwired: 1 in, 2 out]
                      }
                      frame #1 {
                        n232 = call "GVSSearch Matrix Element.vi"("element"=w496, "index (row)"=0, "matrix in"=w497) -> ("index of element"=w495:i32)  [unwired: 8 in]
                        n233 = case shown="True" w501 {
                          tunnel: w495 -> [w504 w526]
                          tunnel: w497 -> [w512 w534]
                          tunnel: w500 -> [w521 w543]
                          tunnel: w499 -> [w520 w542]
                          tunnel: w494 -> [w518 w540]
                          tunnel: [w517 w539] -> w493
                          frame True {
                            n234 = Index Array(array=w512, index (row)=2, index (col)=w504) -> (element=w515:i32)
                            n235 = call "GVSSearch Matrix Element.vi"("element"=w515, "index (row)"=0, "matrix in"=w512) -> ("index of element"=w513:i32)  [unwired: 8 in]
                            n236 = local read "sp_mUp_ypos"() -> (w508:i32)
                            n237 = local read "sp_mUp_hei"() -> (w523:i32)
                            n238 = local read "sp_mUp_xpos"() -> (w506:i32)
                            n239 = Add(x=w508, y=w523) -> (x+y=w503:i32)
                            n240 = Index Array(array=w512, index (row)=5, index (col)=w513) -> (element=w510:i32)
                            n241 = Replace Array Subset(array=w512, new element #1=w510, index (row) #1=5 ("disabled index (row)"), index (col) #1=w504, new element #2=w508, index (row) #2=6 ("disabled index (row)"), index (col) #2=w504, new element #3=w506, index (row) #3=7 ("disabled index (row)"), index (col) #3=w504, new element #4=w503, index (row) #4=8 ("disabled index (row)"), index (col) #4=w504) -> (w502:i32[][])
                            n242 = Bundle By Name(cluster=w521, "Spliter_matrix"=w502) -> (w522:T1)
                            n243 = Replace Array Subset(array=w518, new element=w522, index=w520) -> (w517:T1[])
                          }
                          frame False {
                            n244 = Index Array(array=w534, index (row)=2, index (col)=w526) -> (element=w537:i32)
                            n245 = call "GVSSearch Matrix Element.vi"("element"=w537, "index (row)"=0, "matrix in"=w534) -> ("index of element"=w535:i32)  [unwired: 8 in]
                            n246 = local read "sp_mUp_ypos"() -> (w530:i32)
                            n247 = local read "sp_mUp_xpos"() -> (w546:i32)
                            n248 = local read "sp_mUp_wid"() -> (w545:i32)
                            n249 = local read "sp_mUp_hei"() -> (w547:i32)
                            n250 = Add(x=w546, y=w545) -> (x+y=w532:i32)
                            n251 = Add(x=w530, y=w547) -> (x+y=w525:i32)
                            n252 = Index Array(array=w534, index (row)=7, index (col)=w535) -> (element=w528:i32)
                            n253 = Replace Array Subset(array=w534, new element #1=w532, index (row) #1=5 ("disabled index (row)"), index (col) #1=w526, new element #2=w530, index (row) #2=6 ("disabled index (row)"), index (col) #2=w526, new element #3=w528, index (row) #3=7 ("disabled index (row)"), index (col) #3=w526, new element #4=w525, index (row) #4=8 ("disabled index (row)"), index (col) #4=w526) -> (w524:i32[][])
                            n254 = Bundle By Name(cluster=w543, "Spliter_matrix"=w524) -> (w544:T1)
                            n255 = Replace Array Subset(array=w540, new element=w544, index=w542) -> (w539:T1[])
                          }
                        }
                      }
                    }
                  }
                }
              }
            }
          }
          frame #1 {
            n256 = Index Array(array=w548, index=w551) -> (element=w552:T1)
            n257 = Unbundle By Name(w552) -> ("Spliter_matrix"=w549:i32[][], "Panel_matrix"=w550:i32[][])
            n258 = while {
              shift-right: [w557] -> _
              shift-left: -1 -> [w560]
              tunnel: w556 -> [w558]
              tunnel: w555 -> [w567]
              tunnel: w554 -> [w566]
              tunnel: w550 -> [w562]
              tunnel: w549 -> [w563]
              stop <- w565 stop-if-true
              n259 = Increment(x=w560) -> (x+1=w559:i32)
              n260 = call "GVSSearch Matrix Element.vi"("start index"=w559, "element"=w558, "index (row)"=0, "matrix in"=w562) -> ("index of element"=w557:i32)  [unwired: 7 in]
              n261 = Less Than 0?(x=w557) -> (x < 0?=w565:bool)
              n262 = Not(x=w565) -> (.not. x?=w564:bool)
              n263 = case shown="True" w564 {
                tunnel: w557 -> [_ w581]
                tunnel: w567 -> [_ w588]
                tunnel: w566 -> [_ w590]
                tunnel: w558 -> [_ w585]
                tunnel: w563 -> [_ w573]
                tunnel: w562 -> [_ w582]
                frame False {
                }
                frame True {
                  n264 = stacked-sequence {
                    tunnel: w590 -> [w592]
                    tunnel: w585 -> [w593]
                    tunnel: [w592] -> w589
                    frame #0 {
                      n265 = Index Array(array=w592, index=w593) -> (element=w591:refnum<vi>)
                      n266 = property class="Bool"(reference=w591) -> ("Left"=w597:i32, "Top"=w596:i32)  [unwired: 1 in, 2 out]
                      n267 = local write "cur_sp_xpos"(w597) -> ()
                      n268 = local write "cur_sp_ypos"(w596) -> ()
                      n269 = property class="Bool"(reference=w591) -> ("Height"=w595:u32, "Width"=w594:u32)  [unwired: 1 in, 2 out]
                      n270 = local write "cur_sp_hei"(w595) -> ()
                      n271 = local write "cur_sp_wid"(w594) -> ()
                    }
                  }
                  n272 = Index Array(array=w582, index (row) #1=1 ("index (row)"), index (col) #1=w581, index (row) #2=2 ("index (row)"), index (col) #2=w581) -> (element #1=w580:i32, element #2=w579:i32)
                  n273 = Index Array(array=w588, index=w580) -> (element=w587:refnum<vi>)
                  n274 = call "GVSSearch Matrix Element.vi"("element"=w585, "index (row)"=0, "matrix in"=w573) -> ("index of element"=w574:i32)  [unwired: 8 in]
                  n275 = Index Array(array=w573, index (row) #1=5 ("index (row)"), index (col) #1=w574, index (row) #2=6 ("index (row)"), index (col) #2=w574, index (row) #3=7 ("index (row)"), index (col) #3=w574, index (row) #4=8 ("index (row)"), index (col) #4=w574) -> (element #1=w572:i32, element #2=w571:i32, element #3=w570:i32, element #4=w569:i32)
                  n276 = global read "GVSNew View Global.vi" "panel_offset"() -> (w568:i32)
                  n277 = case shown="4" w579 {
                    tunnel: w572 -> [_ w605 _ w622 w626]
                    tunnel: w571 -> [_ w606 w614 w619 _]
                    tunnel: w570 -> [_ _ w613 _ _]
                    tunnel: w569 -> [_ _ _ _ w630]
                    tunnel: w589 -> [_ _ _ _ _]
                    tunnel: w587 -> [_ w601 w617 w623 w634]
                    tunnel: w568 -> [_ w598 w607 _ w624]
                    frame 0, Default {
                    }
                    frame 1 {
                      n278 = local read "cur_sp_xpos"() -> (w604:i32)
                      n279 = local read "cur_sp_hei"() -> (w602:i32)
                      n280 = Subtract(x=w605, y=w598) -> (x-y=w600:i32)
                      n281 = Subtract(x=w604, y=w605) -> (x-y=w603:i32)
                      n282 = Subtract(x=w606, y=w598) -> (x-y=w599:i32)
                      n283 = property class="SubPnl"(reference=w601, "Width"=w603, "Height"=w602, "Left"=w600, "Top"=w599) -> ()  [unwired: 1 in, 2 out]
                    }
                    frame 2 {
                      n284 = local read "cur_sp_xpos"() -> (w616:i32)
                      n285 = local read "cur_sp_wid"() -> (w615:i32)
                      n286 = Add(x=w616, y=w615) -> (x+y=w612:i32)
                      n287 = local read "cur_sp_hei"() -> (w610:i32)
                      n288 = Subtract(x=w613, y=w612) -> (x-y=w611:i32)
                      n289 = Subtract(x=w614, y=w607) -> (x-y=w608:i32)
                      n290 = Subtract(x=w612, y=w607) -> (x-y=w609:i32)
                      n291 = property class="SubPnl"(reference=w617, "Width"=w611, "Height"=w610, "Left"=w609, "Top"=w608) -> ()  [unwired: 1 in, 2 out]
                    }
                    frame 3 {
                      n292 = local read "cur_sp_ypos"() -> (w620:i32)
                      n293 = local read "cur_sp_wid"() -> (w621:i32)
                      n294 = Subtract(x=w620, y=w619) -> (x-y=w618:i32)
                      n295 = property class="SubPnl"(reference=w623, "Width"=w621, "Height"=w618, "Left"=w622, "Top"=w619) -> ()  [unwired: 1 in, 2 out]
                    }
                    frame 4 {
                      n296 = local read "cur_sp_ypos"() -> (w632:i32)
                      n297 = local read "cur_sp_hei"() -> (w631:i32)
                      n298 = Add(x=w632, y=w631) -> (x+y=w629:i32)
                      n299 = local read "cur_sp_wid"() -> (w633:i32)
                      n300 = Subtract(x=w630, y=w629) -> (x-y=w628:i32)
                      n301 = Subtract(x=w626, y=w624) -> (x-y=w627:i32)
                      n302 = Subtract(x=w629, y=w624) -> (x-y=w625:i32)
                      n303 = property class="SubPnl"(reference=w634, "Width"=w633, "Height"=w628, "Left"=w627, "Top"=w625) -> ()  [unwired: 1 in, 2 out]
                    }
                  }
                }
              }
            }
          }
        }
      }
    }
  }
  n304 = global write "GVSNew View Global.vi" "DataView_Global"(w6) -> ()
